vi "IsTheory.vi"(8 "error in (no error)":errorcluster, 10 "VI Refnum":refnum<vi>) -> (0 "error out":errorcluster, 2 "Is Theory?":bool)   [LabVIEW 2019, in "TestSuite.lvclass"]
uses:
  TestSuite.lvclass
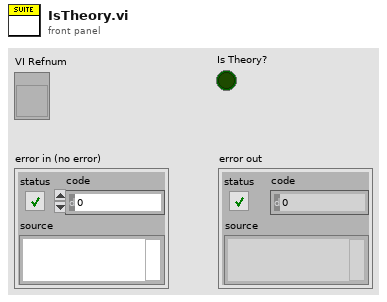
[diagram p1: front panel]
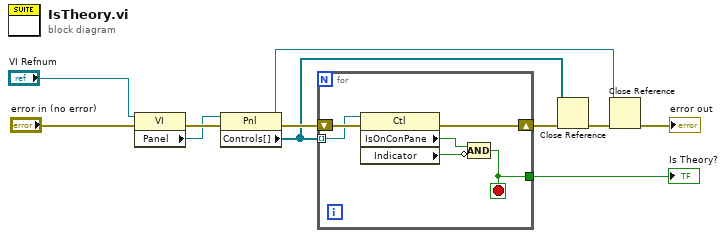
[diagram p0: block diagram]
diagram:
  n1 = property class="VI"(reference="VI Refnum", error in="error in (no error)") -> (error out=w11:errorcluster, "Panel"=w10:refnum<vi>)  [unwired: 1 out]
  n2 = property class="Pnl"(reference=w10, error in=w11) -> (reference out=w8:refnum<vi>, error out=w9:errorcluster, "Controls[]"=w5:refnum<vi>[])
  n3 = for {
    tunnel: w5 -> [w16] mode=indexing
    shift-right: [w15] -> w7
    shift-left: w9 -> [w17]
    tunnel: [w12] -> w3
    stop <- w12 stop-if-true
    n4 = property class="Ctl"(reference=w16, error in=w17) -> (error out=w15:errorcluster, "IsOnConPane"=w13:bool, "Indicator"=w14:bool)  [unwired: 1 out]
    n5 = Compound Arithmetic op=AND(w13, invert w14) -> (w12:bool)
  }
  "Is Theory?" <- w3
  n6 = Close Reference(reference=w5, error in (no error)=w7) -> (error out=w6:errorcluster)
  n7 = Close Reference(reference=w8, error in (no error)=w6) -> (error out=→"error out":errorcluster)
